vi "Transmitter with two channels.vi"() -> ()   [LabVIEW 2019]
doc: "Configures a single device to use two channels for transmission in a synchronous manner."
uses:
  <instrlib>/niUSRP/niUSRP Timestamp.ctl
  <instrlib>/niUSRP/niUSRP Configure Time Start Trigger.vi
  <vilib>/Utility/file.llb/Read From Spreadsheet File (DBL).vi
  <instrlib>/niUSRP/niUSRP Write Tx Data (2D CDB).vi
panel:
  out "Data 2":dbl[](graph)
  in  "Upload Chunk Size 2":i32=100000
  in  "file2 (use dialog)":path=path "C:/Users/Burton/Desktop/软件定义平台/OFDM信号/ZC-64.txt"
  out "Data":dbl[](graph)
  in  "Upload Chunk Size":i32=100000
  in  "file1 (use dialog)":path=path "C:/Users/Burton/Desktop/软件定义平台/OFDM信号/G-64.txt"
  out "error out 2":errorcluster
  in  "Timeout 2":dbl=10.0
  in  "Stop 2":bool
  out "error out":errorcluster
  in  "Tab Control":enum32{"NI-294x/295x/X410", "NI-2900/2901"}(tab)
  in  "Channel 0 Carrier Frequency [Hz]":dbl=2000000000.0 format="%#_6p"
  in  "Channel 1 Carrier Frequency [Hz]":dbl=2000000000.0 format="%#_6p"
  in  "Configuration:IQ Rate":dbl
  in  "Configuration:IQ Rate 2":dbl
  in  "Start Trigger Time":T1={"whole seconds"=1, "fractional seconds"=0.0}
  in  "Channel 1 Active Antenna":string="TX1"
  in  "Channel 0 Active Antenna":string="TX1"
  in  "Channel 1 Gain":dbl=10.0 format="%#_6f"
  in  "Stop":bool
  in  "Device Name":refnum<k15>="192.168.10.2"
  in  "Timeout":dbl=10.0
  in  "Channel 0 Gain":dbl=10.0 format="%#_6f"
  # "For X410 use TX/RX0"
  # "For X410 use TX/RX0"
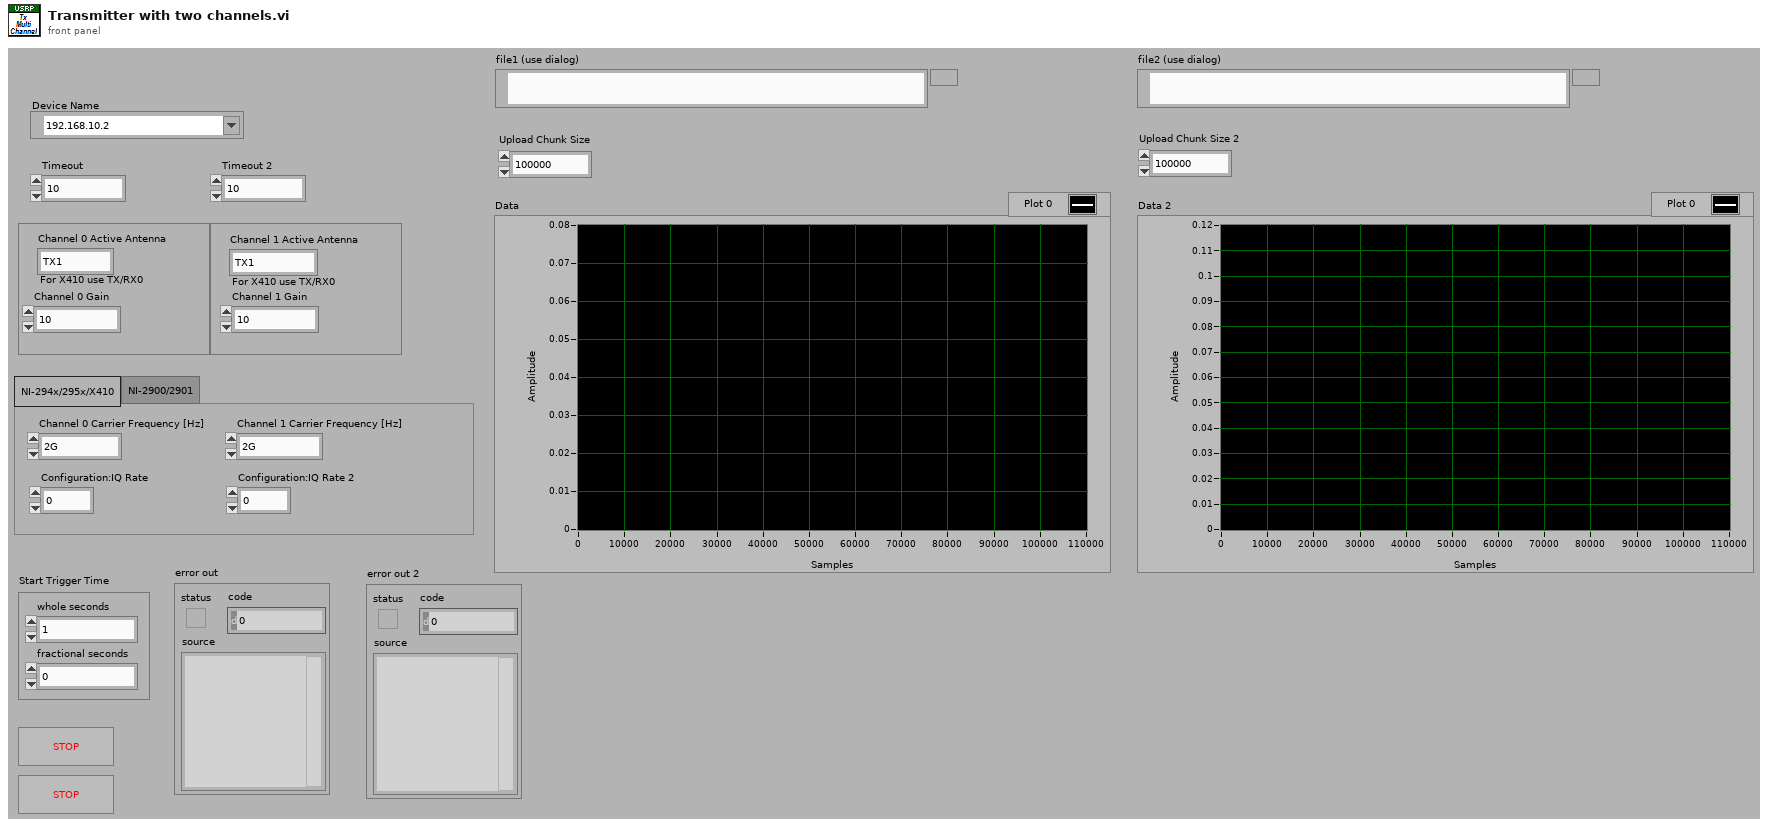
[diagram p1: front panel]
types:
  T1 = typedef "niUSRP Timestamp.ctl" = cluster{"whole seconds":u64, "fractional seconds":dbl}
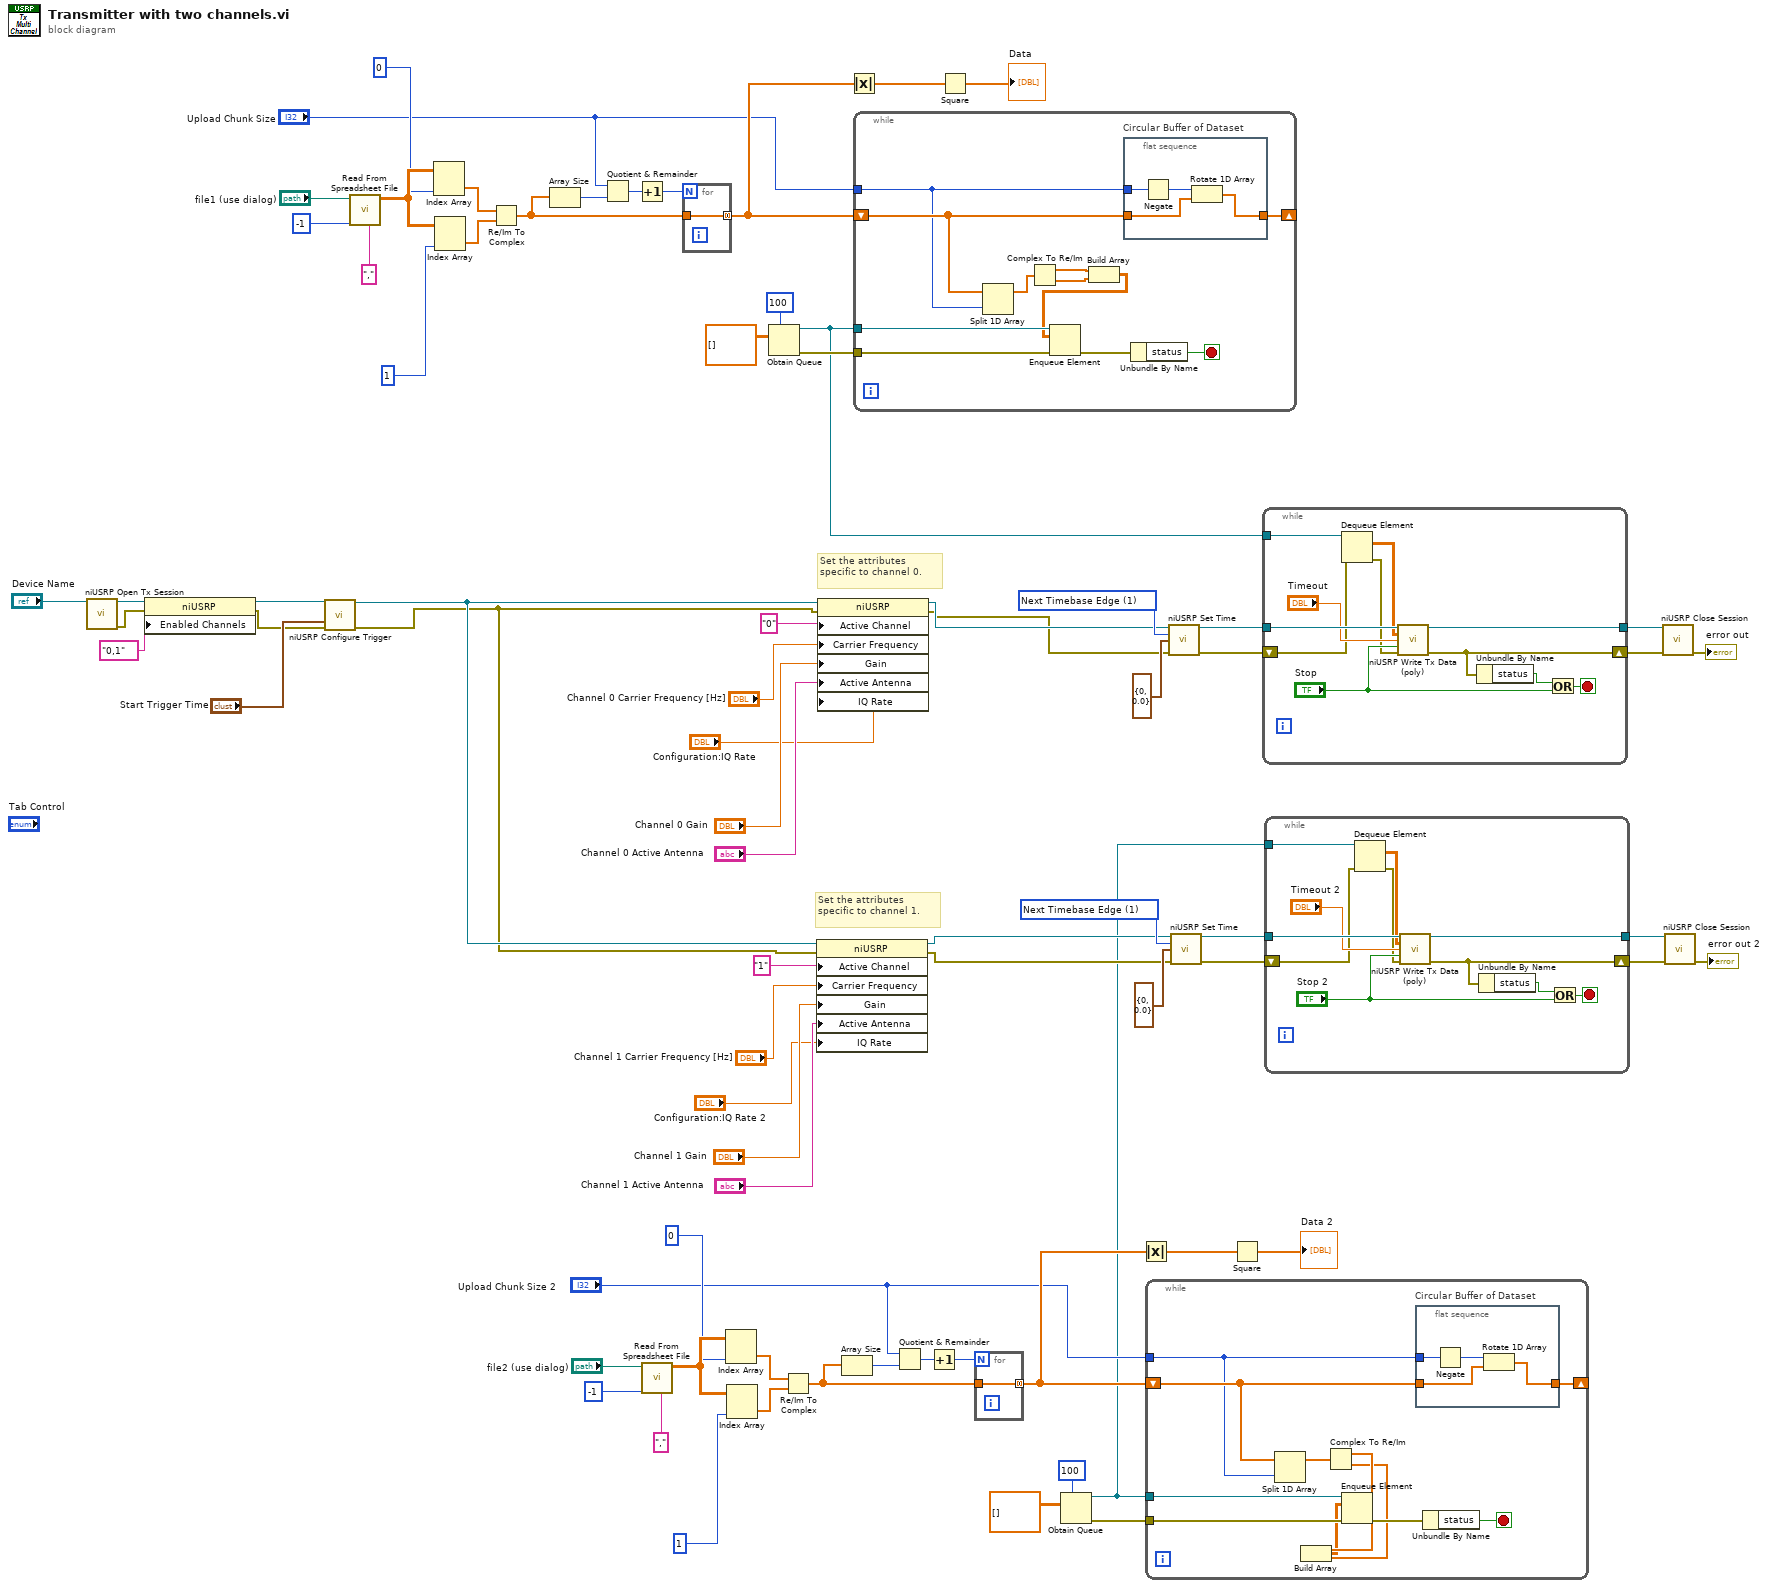
[diagram p0: block diagram]
diagram:
  w52 = 1 items=["Now", "Next Timebase Edge"] ("apply timestamp")
  w66 = 1 items=["Now", "Next Timebase Edge"] ("apply timestamp")
  # "Set the attributes \nspecific to channel 1."
  # "Set the attributes \nspecific to channel 0."
  n1 = call <instrlib>:"niUSRP Open Tx Session.vi"("device names"="Device Name") -> ("session handle out"=w65:refnum<k15>, "error out"=w64:errorcluster)  [unwired: 13 in]
  n2 = property class="niUSRP"(reference=w65, error in=w64, "Enabled Channels"="0,1" ("Configuration:Enabled Channels")) -> (reference out=w63:refnum<k15>, error out=w62:errorcluster)
  n3 = call-poly <instrlib>:"niUSRP Configure Trigger.vi"("session handle"=w63, "start trigger time"="Start Trigger Time", "error in (no error)"=w62) -> ("session handle out"=w50:refnum<k15>, "error out"=w49:errorcluster)  [unwired: 11 in]
  n4 = call-poly <vilib>:"Read From Spreadsheet File.vi"("delimiter (\\t)"="," ("delimiter (\\t)"), "number of rows (all:-1)"=-1, "file path (dialog if empty)"="file1 (use dialog)") -> ("all rows"=w34:dbl[][])  [unwired: 4 in, 4 out]
  n5 = Index Array(array=w34, index (col)=0 ("disabled index (col)")) -> (element=w32:dbl[])  [unwired: 1 in]
  n6 = Index Array(array=w34, index (col)=1 ("disabled index (col)")) -> (element=w33:dbl[])  [unwired: 1 in]
  n7 = Re/Im To Complex(1:w33, 2:w32) -> (0:w28:cdb[])
  n8 = Array Size(array=w28) -> (size(s)=w27:i32)
  n9 = Quotient & Remainder(x="Upload Chunk Size", y=w27) -> (floor(x/y)=w25:i32)  [unwired: 1 out]
  n10 = Increment(x=w25) -> (x+1=w24:i32)
  n11 = call-poly <vilib>:"Read From Spreadsheet File.vi"("delimiter (\\t)"="," ("delimiter (\\t)"), "number of rows (all:-1)"=-1, "file path (dialog if empty)"="file2 (use dialog)") -> ("all rows"=w15:dbl[][])  [unwired: 4 in, 4 out]
  n12 = for {
    N: w24 -> [_]
    tunnel: [w78] -> w29 mode=concatenating
    tunnel: w28 -> [w78]
  }
  n13 = Index Array(array=w15, index (col)=0 ("disabled index (col)")) -> (element=w13:dbl[])  [unwired: 1 in]
  n14 = Index Array(array=w15, index (col)=1 ("disabled index (col)")) -> (element=w14:dbl[])  [unwired: 1 in]
  n15 = Obtain Queue(max queue size (-1, unlimited)=100, element data type=dbl[][] [] ("元素数据类型")) -> (queue out=w23:refnum<queue>, error out=w37:errorcluster)  [unwired: 3 in, 1 out]
  n16 = Re/Im To Complex(1:w14, 2:w13) -> (0:w9:cdb[])
  n17 = property class="niUSRP"(reference=w50, error in=w49, "Active Channel"="1", "Carrier Frequency"="Channel 1 Carrier Frequency [Hz]", "Gain"="Channel 1 Gain", "Active Antenna"="Channel 1 Active Antenna", "IQ Rate"="Configuration:IQ Rate 2") -> (reference out=w45:refnum<k15>, error out=w44:errorcluster)
  n18 = property class="niUSRP"(reference=w50, error in=w49, "Active Channel"="0", "Carrier Frequency"="Channel 0 Carrier Frequency [Hz]", "Gain"="Channel 0 Gain", "Active Antenna"="Channel 0 Active Antenna", "IQ Rate"="Configuration:IQ Rate") -> (reference out=w48:refnum<k15>, error out=w43:errorcluster)
  n19 = Array Size(array=w9) -> (size(s)=w8:i32)
  n20 = Absolute Value(x=w29) -> (abs(x)=w38:dbl[])
  n21 = while {
    tunnel: w23 -> [w84]
    tunnel: w37 -> [w83]
    shift-right: [w87] -> _
    shift-left: w29 -> [w86]
    tunnel: "Upload Chunk Size" -> [w85]
    stop <- w89 stop-if-true
    n22 = Split 1D Array(array=w86, index=w85) -> (first subarray=w82:cdb[])  [unwired: 1 out]
    n23 = Complex To Re/Im(x + iy=w82) -> (x=w81:dbl[], y=w80:dbl[])
    n24 = Build Array(w81, w80) -> (w79:dbl[][])
    n25 = Enqueue Element(queue=w84, element=w79, error in (no error)=w83) -> (error out=w88:errorcluster)  [unwired: 1 in, 2 out]
    n26 = flat-sequence "Circular Buffer of Dataset" {
      tunnel: [w93] -> w87
      tunnel: w86 -> [w92]
      tunnel: w85 -> [w90]
      frame #0 {
        n27 = Negate(x=w90) -> (-x=w91:i32)
        n28 = Rotate 1D Array(1:w92, 2:w91) -> (0:w93:cdb[])
      }
    }
    n29 = Unbundle By Name(w88) -> ("status"=w89:bool)
  }
  n30 = Quotient & Remainder(x="Upload Chunk Size 2", y=w8) -> (floor(x/y)=w6:i32)  [unwired: 1 out]
  n31 = Increment(x=w6) -> (x+1=w5:i32)
  n32 = Square(x=w38) -> (x^2=→"Data":dbl[])
  n33 = for {
    N: w5 -> [_]
    tunnel: [w94] -> w10 mode=concatenating
    tunnel: w9 -> [w94]
  }
  n34 = Obtain Queue(max queue size (-1, unlimited)=100, element data type=dbl[][] []) -> (queue out=w3:refnum<queue>, error out=w18:errorcluster)  [unwired: 3 in, 1 out]
  n35 = Absolute Value(x=w10) -> (abs(x)=w19:dbl[])
  n36 = while {
    tunnel: w3 -> [w100]
    tunnel: w18 -> [w99]
    shift-right: [w103] -> _
    shift-left: w10 -> [w102]
    tunnel: "Upload Chunk Size 2" -> [w101]
    stop <- w105 stop-if-true
    n37 = Split 1D Array(array=w102, index=w101) -> (first subarray=w98:cdb[])  [unwired: 1 out]
    n38 = Complex To Re/Im(x + iy=w98) -> (x=w97:dbl[], y=w96:dbl[])
    n39 = Build Array(w97, w96) -> (w95:dbl[][])
    n40 = Enqueue Element(queue=w100, element=w95, error in (no error)=w99) -> (error out=w104:errorcluster)  [unwired: 1 in, 2 out]
    n41 = flat-sequence "Circular Buffer of Dataset" {
      tunnel: [w109] -> w103
      tunnel: w102 -> [w108]
      tunnel: w101 -> [w106]
      frame #0 {
        n42 = Negate(x=w106) -> (-x=w107:i32)
        n43 = Rotate 1D Array(1:w108, 2:w107) -> (0:w109:cdb[])
      }
    }
    n44 = Unbundle By Name(w104) -> ("status"=w105:bool)
  }
  n45 = call <instrlib>:"niUSRP Set Time.vi"("session handle"=w48, "apply timestamp"=w66, "timestamp"=T1 {"whole seconds"=0, "fractional seconds"=0.0}, "error in (no error)"=w43) -> ("session handle out"=w68:refnum<k15>, "error out"=w42:errorcluster)  [unwired: 10 in]
  n46 = call <instrlib>:"niUSRP Set Time.vi"("session handle"=w45, "apply timestamp"=w52, "timestamp"=T1 {"whole seconds"=0, "fractional seconds"=0.0}, "error in (no error)"=w44) -> ("session handle out"=w54:refnum<k15>, "error out"=w4:errorcluster)  [unwired: 10 in]
  n47 = Square(x=w19) -> (x^2=→"Data 2":dbl[])
  n48 = while {
    tunnel: w68 -> [w120]
    tunnel: [w118] -> w74
    shift-right: [w117] -> w73
    shift-left: w42 -> [w113]
    tunnel: w23 -> [w111]
    stop <- w116 stop-if-true
    n49 = Dequeue Element(queue=w111, error in (no error)=w113) -> (element=w110:dbl[][], error out=w112:errorcluster)  [unwired: 1 in, 2 out]
    n50 = call-poly <instrlib>:"niUSRP Write Tx Data (poly).vi"("session handle"=w120, "data"=w110, "timeout"="Timeout", "end of data?"="Stop", "error in (no error)"=w112) -> ("session handle out"=w118:refnum<k15>, "error out"=w117:errorcluster)  [unwired: 9 in]
    n51 = Unbundle By Name(w117) -> ("status"=w115:bool)
    n52 = Or(x=w115, y="Stop") -> (x .or. y?=w116:bool)
  }
  n53 = while {
    tunnel: w54 -> [w131]
    tunnel: [w129] -> w56
    shift-right: [w128] -> w55
    shift-left: w4 -> [w124]
    tunnel: w3 -> [w122]
    stop <- w127 stop-if-true
    n54 = Dequeue Element(queue=w122, error in (no error)=w124) -> (element=w121:dbl[][], error out=w123:errorcluster)  [unwired: 1 in, 2 out]
    n55 = call-poly <instrlib>:"niUSRP Write Tx Data (poly).vi"("session handle"=w131, "data"=w121, "timeout"="Timeout 2", "end of data?"="Stop 2", "error in (no error)"=w123) -> ("session handle out"=w129:refnum<k15>, "error out"=w128:errorcluster)  [unwired: 9 in]
    n56 = Unbundle By Name(w128) -> ("status"=w126:bool)
    n57 = Or(x=w126, y="Stop 2") -> (x .or. y?=w127:bool)
  }
  n58 = call <instrlib>:"niUSRP Close Session.vi"("session handle"=w74, "error in (no error)"=w73) -> ("error out"=→"error out":errorcluster)  [unwired: 13 in]
  n59 = call <instrlib>:"niUSRP Close Session.vi"("session handle"=w56, "error in (no error)"=w55) -> ("error out"=→"error out 2":errorcluster)  [unwired: 13 in]
